vi "20170321-lecture2-Cluster.vi"() -> ()   [LabVIEW 2014]
panel:
  out "Cluster 3":T1
  out "String 3":string
  out "Boolean 2":bool
  out "Numeric 2":dbl
  out "String 2":string
  out "Numeric":dbl
  out "String":string
  out "Boolean":bool
  in  "Cluster":T1
  # "Unbundle by Name"
  # "Unbundle"
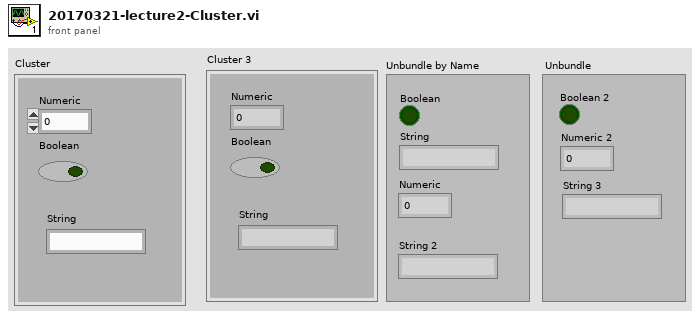
[diagram p1: front panel]
types:
  T1 = cluster{"Boolean":bool, "Numeric":dbl, "String":string}
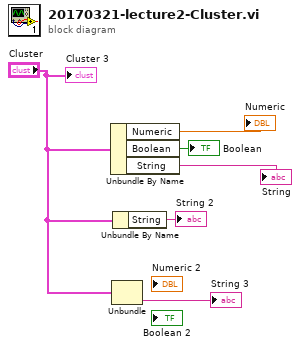
[diagram p0: block diagram]
diagram:
  n1 = Unbundle By Name("Cluster") -> ("Numeric"=→"Numeric":dbl, "Boolean"=→"Boolean":bool, "String"=→"String":string)
  n2 = Unbundle("Cluster") -> ("String"=→"String 3":string)  [unwired: 2 out]
  n3 = Unbundle By Name("Cluster") -> ("String"=→"String 2":string)
  "Cluster 3" <- "Cluster"
